vi "_Smooth Data.vi"(7 "Data In":dbl[](array[numeric])) -> (3 "Data Out":dbl[](array[numeric]))   [LabVIEW 2015]
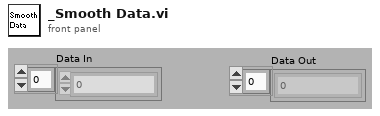
[diagram p1: front panel]
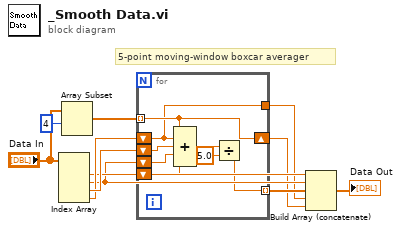
[diagram p0: block diagram]
diagram:
  # "5-point moving-window boxcar averager"
  n1 = Index Array(array="Data In") -> (element #1=w7:dbl, element #2=w5:dbl, element #3=w9:dbl, element #4=w8:dbl)  [unwired: 4 in]
  n2 = Array Subset(array="Data In", index=4) -> (w10:dbl[])  [unwired: 1 in]
  n3 = for {
    shift-right: [w13] -> w3
    shift-left: w8 -> [w12]
    shift-left: w9 -> [w19]
    shift-left: w5 -> [w18]
    shift-left: w7 -> [w17]
    tunnel: w10 -> [w13] mode=indexing
    tunnel: [w14] -> w6 mode=indexing
    tunnel: [w12] -> w4
    n4 = Compound Arithmetic op=ADD(w13, w12, w19, w18, w17) -> (w16:dbl)
    n5 = Divide(x=w16, y=5.0) -> (x/y=w14:dbl)
  }
  n6 = Build Array (concatenate)(w7, w5, w6, w4, w3) -> (→"Data Out":dbl[])
